vi "randomRange.vi"(10 "Minimum value":dbl, 11 "Range":dbl) -> (3 "Random":i32)   [LabVIEW 2017]
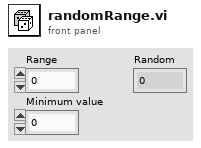
[diagram p1: front panel]
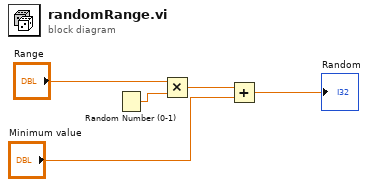
[diagram p0: block diagram]
diagram:
  n1 = Random Number (0-1)() -> (number: 0 to 1=w5:dbl)
  n2 = Multiply(x="Range", y=w5) -> (x*y=w4:dbl)
  n3 = Add(x=w4, y="Minimum value") -> (x+y=→"Random":dbl)
